vi "Back.vi"(8 "error in (no error)":errorcluster, 11 "Steps in":refnum<class "Steps.lvclass">) -> (0 "error out":errorcluster, 1 "Step Number":i32, 2 "Reached Start?":bool, 3 "Steps out":refnum<class "Steps.lvclass">)   [LabVIEW 2015, in "Steps.lvclass"]
doc: "<b> </b> <b> </b>\n©2016 Q Software Innovations, LLC (QSI)\nwritten by Quentin Alldredge\nproduced in LabVIEW 2015\n\nsupport@qsoftwareinnovations.com\nwww.qsoftwareinnovations.com\n\nAll rights reserved.\n\nRedistribution and use in source and binary forms, with or without modification, are permitted provided that the following conditions are met:\n\n * Redistributions of source code must retain the above copyright notice, this list of conditions and the following disclaimer.\n * Redistributions in binary form must reproduce the above copyright notice, this list of conditions and the following disclaimer in the documentation and/or other materials provided with the distribution.\n * Neither the name of Q Software Innovations, LLC. nor the names of its contributors may be used to endorse or promote products derived from this software without specific prior written permission.\n\nTHIS SOFTWARE IS PROVIDED BY THE COPYRIGHT HOLDERS AND CONTRIBUTORS \"AS IS\" AND ANY EXPRESS OR IMPLIED WARRANTIES, INCLUDING, BUT NOT LIMITED TO, THE IMPLIED WARRANTIES OF MERCHANTABILITY AND FITNESS FOR A PARTICULAR PURPOSE ARE DISCLAIMED. IN NO EVENT SHALL THE COPYRIGHT OWNER OR CONTRIBUTORS BE LIABLE FOR ANY DIRECT, INDIRECT, INCIDENTAL, SPECIAL, EXEMPLARY, OR CONSEQUENTIAL DAMAGES (INCLUDING, BUT NOT LIMITED TO, PROCUREMENT OF SUBSTITUTE GOODS OR SERVICES; LOSS OF USE, DATA, OR PROFITS; OR BUSINESS INTERRUPTION) HOWEVER CAUSED AND ON ANY THEORY OF LIABILITY, WHETHER IN CONTRACT, STRICT LIABILITY, OR TORT (INCLUDING NEGLIGENCE OR OTHERWISE) ARISING IN ANY WAY OUT OF THE USE OF THIS SOFTWARE, EVEN IF ADVISED OF THE POSSIBILITY OF SUCH DAMAGE."
uses:
  Steps.lvclass
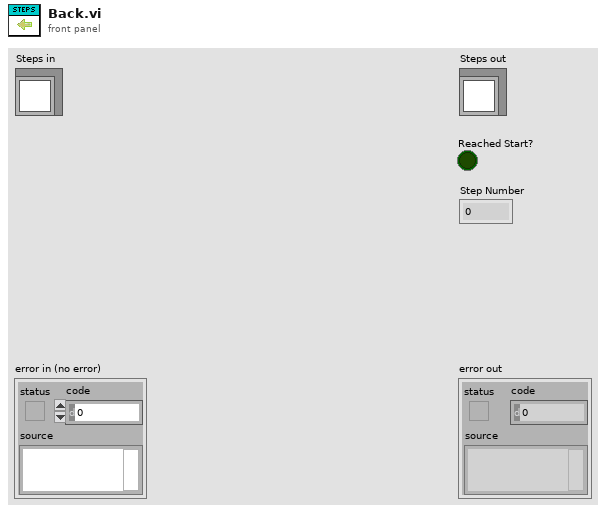
[diagram p1: front panel]
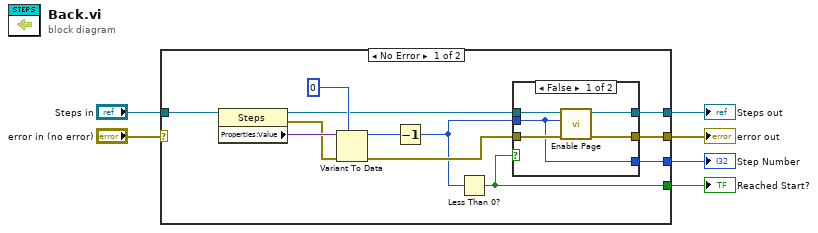
[diagram p0: block diagram]
diagram:
  n1 = case shown="No Error" "error in (no error)" {
    selector: "error in (no error)" -> [_ w28]
    tunnel: [w9 w28] -> w5
    tunnel: [w14 w27] -> w3
    tunnel: "Steps in" -> [w18 w27]
    tunnel: [w11 _] -> w2
    tunnel: [w7 _] -> w1
    frame No Error {
      n2 = property class="Steps"(reference=w18) -> (reference out=w15:refnum<class "Steps.lvclass">, error out=w12:errorcluster, "Properties:Value"=w17:variant)  [unwired: 1 in]
      n3 = Variant To Data(error in=w12, type=0, Variant=w17) -> (data=w13:i32, error out=w10:errorcluster)
      n4 = Decrement(x=w13) -> (x-1=w8:i32)
      n5 = Less Than 0?(x=w8) -> (x < 0?=w11:bool)
      n6 = case shown="False" w11 {
        tunnel: w15 -> [w23 w26]
        tunnel: [w22 w26] -> w14
        tunnel: w8 -> [w19 w24]
        tunnel: w10 -> [w21 w25]
        tunnel: [w20 w25] -> w9
        tunnel: [w19 w24] -> w7
        frame False {
          n7 = call "Enable Page.vi"("error in (no error)"=w21, "Page Index"=w19, "Steps in"=w23) -> ("error out"=w20:errorcluster, "Steps out"=w22:refnum<class "Steps.lvclass">)  [unwired: 7 in]
        }
        frame True {
        }
      }
    }
    frame Error {
    }
  }
  "error out" <- w5
  "Steps out" <- w3
  "Reached Start?" <- w2
  "Step Number" <- w1
